vi "Report Error.vi"(5 "Callchain (T)":bool=TRUE, 7 "Context (None)":string, 8 "error in (no error)":errorcluster, 11 "Vecto in":refnum<class "Vecto.lvclass">) -> (0 "error out":errorcluster, 3 "Vecto out":refnum<class "Vecto.lvclass">)   [LabVIEW 2020, in "Vecto.lvlib" / "Vecto.lvclass"]
uses:
  Vecto.lvclass
  Vecto.lvclass/Vecto.ctl
  EventLoggingService/EventLoggingService.lvclass
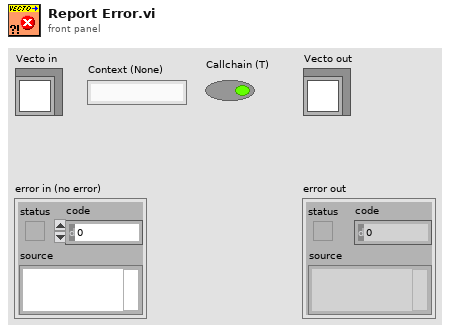
[diagram p1: front panel]
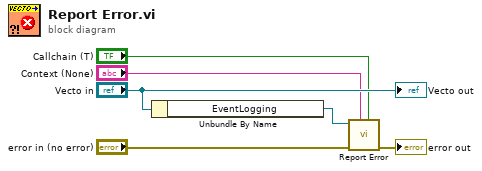
[diagram p0: block diagram]
diagram:
  n1 = Unbundle By Name("Vecto in") -> ("EventLogging"=w5:refnum<class "EventLoggingService.lvclass">)
  n2 = call "Report Error.vi"("Callchain (T)"="Callchain (T)", "Context (None)"="Context (None)", "error in (no error)"="error in (no error)", "EventLoggingService in"=w5) -> ("error out"=→"error out":errorcluster)  [unwired: 6 in, 1 out]
  "Vecto out" <- "Vecto in"
